vi "LB Read Value.vi"(8 "error in (no error)":errorcluster, 11 "LB ref (generic)":refnum<vi>) -> (0 "error out":errorcluster, 2 "Value":i32[](array[numeric]), 3 "LB ref (generic)":refnum<vi>)   [LabVIEW 2020, in "BetterDragAndDrop.lvlib" / "BetterListboxHandle.lvclass"]
uses:
  BetterListboxHandle.lvclass
  <vilib>/Utility/error.llb/Error Cluster From Error Code.vi
  <vilib>/ErrorRing/Error Ring.xnode
  BetterListboxHandle.lvclass/BetterListboxHandle.ctl
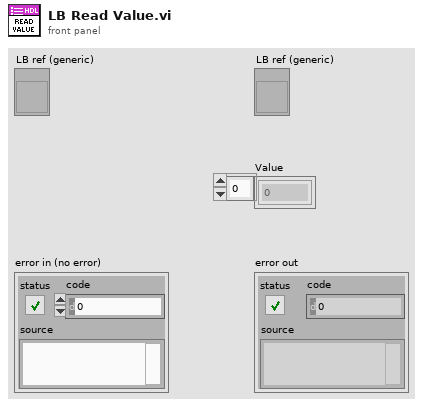
[diagram p1: front panel]
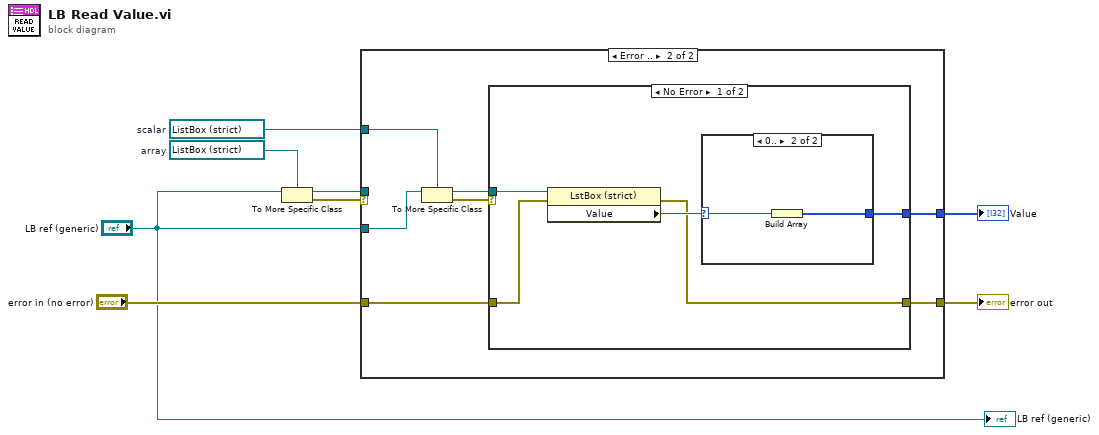
[diagram p0: block diagram]
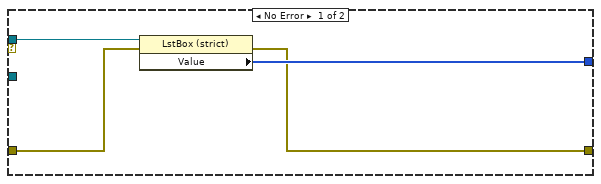
[diagram p2: hidden frame]
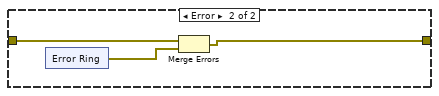
[diagram p4: hidden frame]
diagram:
  w2 = refnum<vi> refnum  # array
  w1 = refnum<vi> refnum  # scalar
  n1 = To More Specific Class(target class=w2, reference="LB ref (generic)") -> (specific class reference=w7:refnum<vi>, error out=w8:errorcluster)  [unwired: 1 in]
  n2 = case shown="Error .." w8 {
    tunnel: w7 -> [w12 _]
    tunnel: "LB ref (generic)" -> [_ w19]
    tunnel: w1 -> [_ w18]
    tunnel: "error in (no error)" -> [w10 w15]
    tunnel: [w9 w14] -> w5
    tunnel: [w11 w13] -> w4
    frame No Error {
      n3 = property class="LstBox (strict)"(reference=w12, error in=w10) -> (error out=w9:errorcluster, "Value"=w11:i32[])  [unwired: 1 out]
    }
    frame Error {
      n4 = To More Specific Class(target class=w18, reference=w19) -> (specific class reference=w16:refnum<vi>, error out=w17:errorcluster)  [unwired: 1 in]
      n5 = case shown="No Error" w17 {
        tunnel: w16 -> [w24 _]
        tunnel: w15 -> [w21 w28]
        tunnel: [w20 w27] -> w14
        tunnel: [w22 _] -> w13
        frame No Error {
          n6 = property class="LstBox (strict)"(reference=w24, error in=w21) -> (error out=w20:errorcluster, "Value"=w23:i32)  [unwired: 1 out]
          n7 = case shown="0.." w23 {
            selector: w23 -> [_ w26]
            tunnel: [_ w25] -> w22
            frame Default {
            }
            frame 0.. {
              n8 = Build Array(w26) -> (w25:i32[])
            }
          }
        }
        frame Error {
          n9 = xnode "Error Ring"() -> ("error out"=w29:errorcluster)
          n10 = Merge Errors(w28, w29) -> (w27:errorcluster)
        }
      }
    }
  }
  "error out" <- w5
  "Value" <- w4
  "LB ref (generic)" <- "LB ref (generic)"
